vi "vacuum.vi"(8 "error in (no error)":errorcluster, 10 "Vacuum Setting (0000)":i64 min=0 max=1000 step=1 format="%04.0f", 11 "Ultimus V in":refnum<class "Ultimus V2.lvclass">) -> (0 "error out":errorcluster, 3 "Ultimus V out":refnum<class "Ultimus V2.lvclass">)   [LabVIEW 2016, in "Ultimus V2.lvclass"]
uses:
  Ultimus V2.lvclass
  Ultimus V2.lvclass/Ultimus V2.ctl
  Drivers/EFD Ultimus V/EFD Ultimus V.lvlib
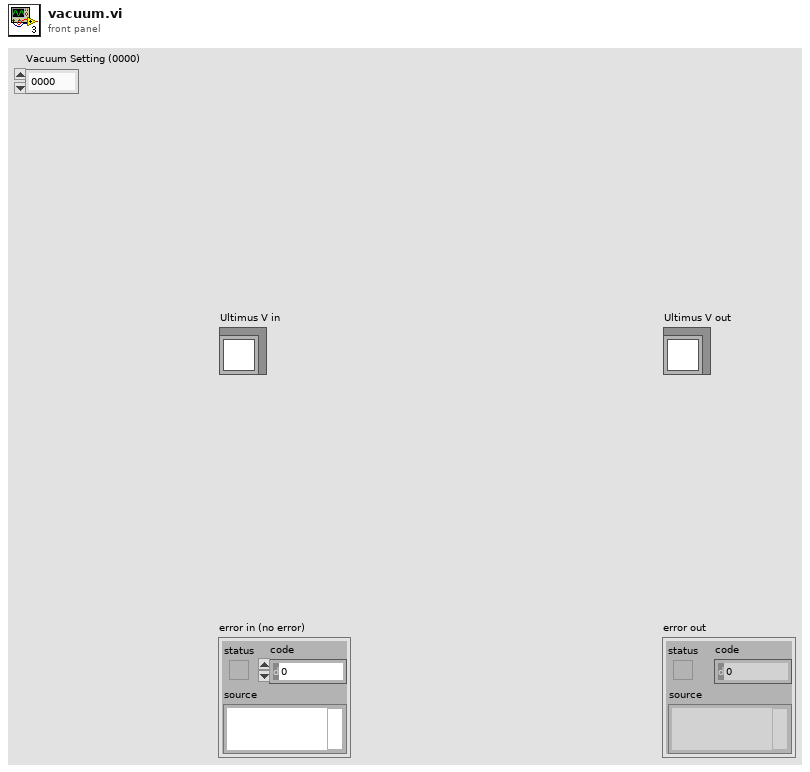
[diagram p1: front panel]
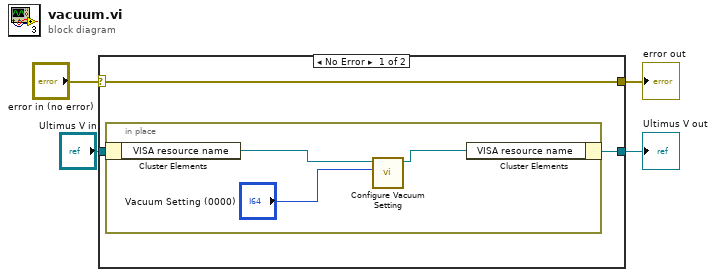
[diagram p0: block diagram]
diagram:
  n1 = case shown="No Error" "error in (no error)" {
    selector: "error in (no error)" -> [w7 w12]
    tunnel: "Ultimus V in" -> [w6 w11]
    tunnel: [w5 w11] -> w3
    tunnel: [w7 w12] -> w1
    frame No Error {
      n2 = in-place {
        n3 = in-place-cluster #1(w6) -> ("VISA resource name"=w10:refnum<visa-resource-name>)
        n4 = call "Configure Vacuum Setting.vi"("Vacuum Setting (0000)"="Vacuum Setting (0000)", "VISA resource name"=w10) -> ("VISA resource name out"=w9:refnum<visa-resource-name>)  [unwired: 8 in, 1 out]
        n5 = in-place-cluster #1("VISA resource name"=w9) -> (w5:refnum<class "Ultimus V2.lvclass">)
      }
    }
    frame Error {
    }
  }
  "error out" <- w1
  "Ultimus V out" <- w3
